vi "FileInfo.vi"() -> ()   [LabVIEW 2017]
panel:
  out "FileInfo":T1 {"strFilePath" format="%x"}
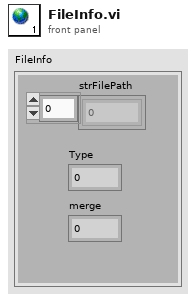
[diagram p1: front panel]
types:
  T1 = cluster{"strFilePath":i8[], "Type":u8, "merge":u8}
diagram:
